vi "1stHiddenLayerANN.vi"(11 "Input":sgl[](array[numeric])=[0.0, 0.0, 0.0, 0.0, 0.0, 0.0, 0.0, 0.0]) -> (3 "1stHiddenOut":sgl[](array[numeric]))   [LabVIEW 2020]
uses:
  <vilib>/rvi/Memory/Memory_Emulation/nirvimemoryFastEmulation.vi
  <vilib>/rvi/Memory/Memory_Emulation/nirvimemoryEmulation.vi
  <vilib>/rvi/Emulation/niFpgaEmulationIsFPGAContextNoSignature.vi
  <vilib>/rvi/DataTransferAndStorage/Container/Common/niFpgaContainerGetUniqueNameForEmu.vi
  <vilib>/rvi/Emulation/niFpgaProcessEmulError.vi
  <vilib>/rvi/Emulation/niFpgaSctlEmulationGetInTimedLoop.vi
  <vilib>/rvi/errors/nirviReportUnexpectedCaseInternalError (U32).vi
  <vilib>/rvi/DataTransferAndStorage/Container/XNode/niFpgaContainer.xnode
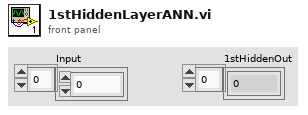
[diagram p1: front panel]
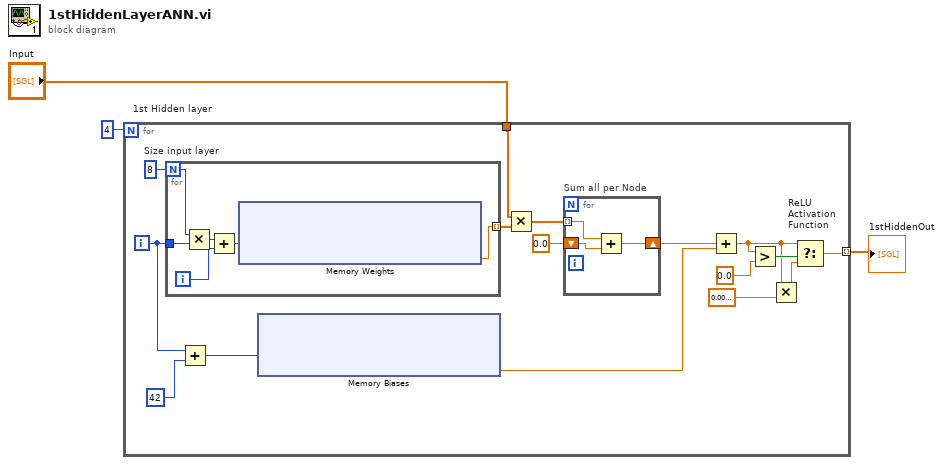
[diagram p0: block diagram]
diagram:
  w1 = 4  # 1st Hidden layer
  n1 = for {
    N: w1 -> [_]
    tunnel: "Input" -> [w19]
    tunnel: [w8] -> w3 mode=indexing
    i -> [w14]
    w15 = 8  # Size input layer
    n2 = for {
      N: w15 -> [w23]
      tunnel: w14 -> [w24]
      tunnel: [w25] -> w18 mode=indexing
      i -> [w21]
      n3 = Multiply(x=w23, y=w24) -> (x*y=w22:i32)
      n4 = Add(x=w22, y=w21) -> (x+y=w20:i32)
      n5 = xnode "Memory Weights"("Address"=w20) -> ("Data"=w25:sgl)  [unwired: 1 in, 1 out]
    }
    n6 = Add(x=w14, y=42) -> (x+y=w13:i32)
    n7 = xnode "Memory Biases"("Address"=w13) -> ("Data"=w7:sgl)  [unwired: 1 in, 1 out]
    n8 = Multiply(x=w19, y=w18) -> (x*y=w17:sgl[])
    n9 = for "Sum all per Node" {
      tunnel: w17 -> [w28] mode=indexing
      shift-right: [w26] -> w11
      shift-left: sgl 0.0 -> [w27]
      n10 = Add(x=w28, y=w27) -> (x+y=w26:sgl)
    }
    n11 = Add(x=w11, y=w7) -> (x+y=w6:sgl)
    n12 = Greater?(x=w6, y=sgl 0.0) -> (0:w10:bool)
    n13 = Multiply(x=w6, y=sgl 0.01) -> (x*y=w5:sgl)
    n14 = Select "ReLU\nActivation\nFunction"(t=w6, s=w10, f=w5) -> (s? t:f=w8:sgl)
  }
  "1stHiddenOut" <- w3
